vi "PSVCH_Caculate Thread.vi"() -> ()   [LabVIEW 2016]
uses:
  ShareLib/Formula/Ctrls/PSFormula_FOR_Formula Node.ctl
  ShareLib/Formula/Ctrls/PSFormula_FOR_Formula Step.ctl
  ShareLib/Formula/Ctrls/PSFormula_FOR_Formula Para.ctl
  ShareLib/Formula/Ctrls/PSFormula_FOR_Formula MidVar Data.ctl
  Ctrls/PSVCH_VarList.ctl
  <vilib>/Platform/TimedLoop/XDataNode/timing_clust.ctl
  <vilib>/Platform/TimedLoop/XDataNode/nitl_modes.ctl
  <vilib>/Platform/TimedLoop/XDataNode/wakeup.ctl
  <vilib>/Platform/TimedLoop/TimeConversion.llb/rt-timestamp-to-milliseconds.vi
  <vilib>/Pansino Software/LabVIEW Architecture/Queue Management/PSARC_Queue Insert Element.vi
  <vilib>/Platform/TimedLoop/XDataNode/XDataNode.xnode
  <vilib>/Platform/TimedLoop/XDataNode/XDNodeRunTimeDep.lvlib
  <vilib>/measure/NI_MABase.lvlib
panel:
  in  "Parameter":variant
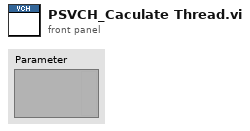
[diagram p1: front panel]
types:
  T1 = typedef "PSFormula_FOR_Formula Node.ctl" = cluster{"Formula Steps":T2[], "MidVar List":T4}
  T2 = typedef "PSFormula_FOR_Formula Step.ctl" = cluster{"Formula Calc":string, "Para":T3[], "Result Var":string, "Result Var Type":string}
  T3 = typedef "PSFormula_FOR_Formula Para.ctl" = cluster{"Para Index":i32, "Tag":string, "Type":string, "Label":string, "Data":variant}
  T4 = typedef "PSFormula_FOR_Formula MidVar Data.ctl" = cluster{"Names":string[], "Types":string[], "Values":variant[]}
  T5 = typedef "PSVCH_VarList.ctl" = cluster{"Tag[]":string[], "Type[]":string[], "Value[]":variant[], "ai[]":string[]}
  T6 = cluster{"Q_High Name":string, "字符串":string, "t0":timestamp, "Time":i64, "Exit":refnum<notifier>, "Dpl":refnum<queue>, "TDMS Ref":refnum<notifier>, "Save":refnum<notifier>, "Formula Node":T1, "VarList":T5, "布尔":bool, "字符串":string, "字符串":string}
  T7 = typedef "XDNodeRunTimeDep.lvlib/timing_clust.ctl" = cluster{"Expected End [f-1]":u64, "Actual End [f-1]":u64, "Finished Late? [f-1]":bool, "Expected End [i-1]":u64, "Actual End [i-1]":u64, "Finished Late? [i-1]":bool, "Expected Start [i]":u64, "Actual Start [i]":u64, "Expected Start [f]":u64, "Actual Start [f]":u64, "Source Name":string, "Structure Name":string, "Period":i64, "Deadline":i64, "Offset":i64, "Start":i64, "Priority":i32, "Timeout":i32, "Mode":T8, "Wakeup Reason":T9, "Error":errorcluster, "Source Type":string, "Secondary Source Type":string, "Global End Time":u64, "Global Start Time":u64, "Frame Duration":u64, "Iteration Duration":u64, "Assigned CPU":i32, "I/O Scan Engine Mode":u32}
  T8 = typedef "XDNodeRunTimeDep.lvlib/nitl_modes.ctl" = enum32{"No Change", "Process missed periods, maintain original phase", "Discard missed periods, maintain original phase", "Process missed periods, ignore original phase", "Discard missed periods, ignore original phase"}
  T9 = typedef "XDNodeRunTimeDep.lvlib/wakeup.ctl" = enum32{"Normal", "Aborted", "Asynchronous wakeup", "Timing source error", "Timed loop error", "Timeout"}
  T10 = cluster{"ai[]":string[], "Type[]":string[], "Value[]":variant[]}
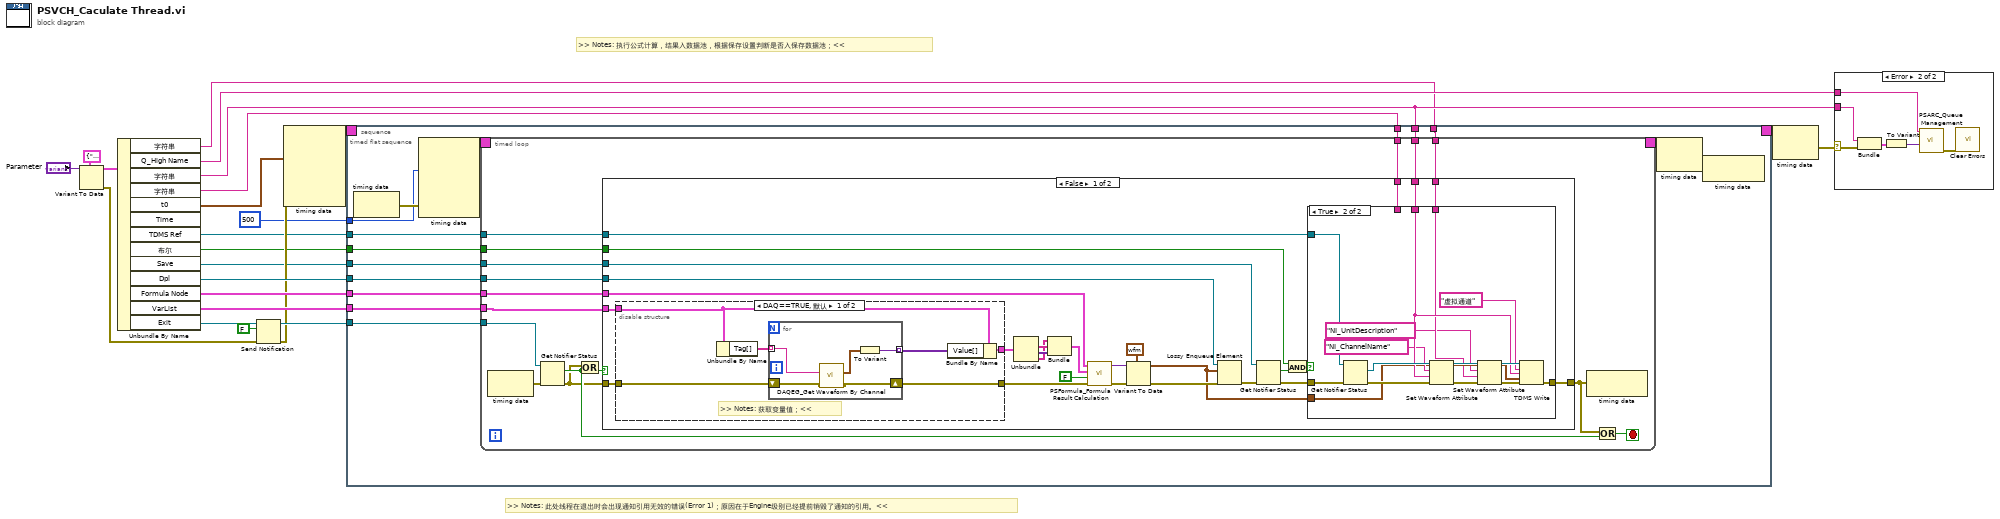
[diagram p0: block diagram]
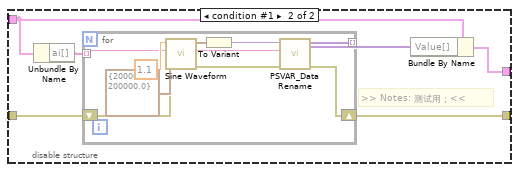
[diagram p3: hidden frame]
diagram:
  # ">> Notes: 此处线程在退出时会出现通知引用无效的错误(Error 1)；原因在于Engine级别已经提前销毁了通知的引用。<<"
  # ">> Notes: 执行公式计算，结果入数据池，根据保存设置判断是否入保存数据池；<<"
  n1 = Variant To Data(type=T6 {"Q_High Name"="", "字符串"="", "t0"=timestamp(0 s since 1904-01-01), "Time"=0, "Exit"=refnum, "Dpl"=refnum, "TDMS Ref"=refnum, "Save"=refnum, "Formula Node"={"Formula Steps"=[], "MidVar List"={"Names"=[], "Types"=[], "Values"=[]}}, "VarList"={"Tag[]"=[], "Type[]"=[], "Value[]"=[], "ai[]"=[]}, "布尔"=FALSE, "字符串"="", "字符串"=""} ("簇"), Variant="Parameter") -> (data=w23:T6, error out=w11:errorcluster)  [unwired: 1 in]
  n2 = Unbundle By Name(w23) -> ("字符串"=w3:string, "Q_High Name"=w21:string, "字符串"=w6:string, "字符串"=w4:string, "t0"=w14:timestamp, "TDMS Ref"=w8:refnum<notifier>, "布尔"=w5:bool, "Save"=w7:refnum<notifier>, "Dpl"=w20:refnum<queue>, "Formula Node"=w19:T1, "VarList"=w18:T5, "Exit"=w13:refnum<notifier>)  [unwired: 1 out]
  n3 = Send Notification(notification=FALSE ("通知"), notifier=w13, error in (no error)=w11) -> (notifier out=w12:refnum<notifier>, error out=w9:errorcluster)
  n4 = node-c288(w14, w9) -> (w17:T7)  [unwired: 3 in]
  n5 = timed-sequence {
    timing: w17 -> [_]
    timing-out: [_] -> w16
    tunnel: i64 500 ("Period") -> [w34]
    tunnel: w20 -> [w33]
    tunnel: w19 -> [w32]
    tunnel: w18 -> [w31]
    tunnel: w12 -> [w30]
    tunnel: w8 -> [w29]
    tunnel: w7 -> [w28]
    tunnel: w6 -> [w27]
    tunnel: w5 -> [w26]
    tunnel: w4 -> [w25]
    tunnel: w3 -> [w24]
    n6 = timed-flat-sequence {
      tunnel: w34 -> [w35]
      tunnel: w33 -> [w47]
      tunnel: w32 -> [w46]
      tunnel: w31 -> [w45]
      tunnel: w30 -> [w43]
      tunnel: w29 -> [w41]
      tunnel: w28 -> [w40]
      tunnel: w27 -> [w39]
      tunnel: w26 -> [w38]
      tunnel: w25 -> [w37]
      tunnel: w24 -> [w36]
      n7 = node-c288() -> (w42:errorcluster)  [unwired: 1 in]
      n8 = node-c288(w35, w42) -> (w49:T7)  [unwired: 3 in]
      n9 = timed-loop {
        timing: w49 -> [_]
        timing-out: [_] -> w48
        tunnel: w47 -> [w63]
        tunnel: w46 -> [w65]
        tunnel: w45 -> [w64]
        tunnel: w43 -> [w61]
        tunnel: w41 -> [w56]
        tunnel: w40 -> [w57]
        tunnel: w39 -> [w55]
        tunnel: w38 -> [w54]
        tunnel: w37 -> [w53]
        tunnel: w36 -> [w50]
        stop <- w58 stop-if-true
        n10 = node-c288() -> (w62:errorcluster)  [unwired: 1 in]
        n11 = Get Notifier Status(notifier=w61, error in (no error)=w62) -> (current notification=w59:bool, error out=w51:errorcluster)  [unwired: 3 out]
        n12 = Or(x=w51, y=w59) -> (x .or. y?=w52:bool)
        n13 = case shown="False" w52 {
          tunnel: w65 -> [w79 _]
          tunnel: w64 -> [w92 _]
          tunnel: [w86 w135] -> w60
          tunnel: w63 -> [w91 _]
          tunnel: w51 -> [w90 w135]
          tunnel: w57 -> [w88 _]
          tunnel: w56 -> [w85 _]
          tunnel: w55 -> [w84 _]
          tunnel: w54 -> [w82 _]
          tunnel: w53 -> [w80 _]
          tunnel: w50 -> [w67 _]
          frame False {
            n14 = disable-structure shown="DAQ==TRUE, 默认" {
              disable-tunnel: w92 -> [w114 w122]
              disable-tunnel: [w113 w125] -> w78
              disable-tunnel: w90 -> [w110 w124]
              disable-tunnel: [w109 w123] -> w71
              frame condition #0 (active) {
                # ">> Notes: 获取变量值；<<"
                n15 = Unbundle By Name(w114) -> ("Tag[]"=w111:string[])
                n16 = for {
                  tunnel: [w119] -> w112 mode=indexing
                  tunnel: w111 -> [w118] mode=indexing
                  shift-right: [w116] -> w109
                  shift-left: w110 -> [w117]
                  n17 = call "DAQEG_Get Waveform By Channel.vi"("error in (no error)"=w117, "DAQ Channel"=w118) -> ("error out"=w116:errorcluster, "waveform"=w115:waveform(dbl))  [unwired: 8 in]
                  n18 = To Variant(anything=w115) -> (Variant=w119:variant)
                }
                n19 = Bundle By Name(cluster=w114, "Value[]"=w112) -> (w113:T5)
              }
              frame condition #1 {
                # ">> Notes: 测试用；<<"
                n20 = Unbundle By Name(w122) -> ("ai[]"=w121:string[])
                n21 = for {
                  tunnel: [w129] -> w120 mode=indexing
                  tunnel: w121 -> [w126] mode=indexing
                  shift-right: [w127] -> w123
                  shift-left: w124 -> [w131]
                  n22 = call <vilib>:"Sine Waveform.vi"("sampling info"=cluster{"Fs":dbl, "#s":dbl} {"Fs"=200000.0, "#s"=200000.0}, "error in (no error)"=w131, "frequency"=1.1) -> ("error out"=w128:errorcluster, "signal out"=w132:waveform(dbl))  [unwired: 7 in]
                  n23 = To Variant(anything=w132) -> (Variant=w130:variant)
                  n24 = call <vilib>:"PSVAR_Data Rename.vi"("error in"=w128, "Name New"=w126, "Data In"=w130) -> ("error out"=w127:errorcluster, "Data Out"=w129:variant)  [unwired: 7 in]
                }
                n25 = Bundle By Name(cluster=w122, "Value[]"=w120) -> (w125:T5)
              }
            }
            n26 = Unbundle(w78) -> ("Type[]"=w77:string[], "Value[]"=w76:variant[], "ai[]"=w72:string[])  [unwired: 1 out]
            n27 = Bundle("ai[]"=w72, "Type[]"=w77, "Value[]"=w76) -> (w75:T10)  [unwired: 1 in]
            n28 = call "PSFormula_Formula Result Calculation.vi"("error in"=w71, "Complex Variable(T)"=FALSE, "Var List"=w75, "Formula Node"=w79) -> ("error out"=w70:errorcluster, "Result Value"=w74:variant)  [unwired: 5 in, 1 out]
            n29 = Variant To Data(error in=w70, type=waveform(dbl) {"t0"=timestamp(0 s since 1904-01-01), "dt"=1.0, "Y"=[]} ("Waveform"), Variant=w74) -> (data=w66:waveform(dbl), error out=w69:errorcluster)
            n30 = Lossy Enqueue Element(queue=w91, element=w66, error in (no error)=w69) -> (error out=w89:errorcluster)  [unwired: 3 out]
            n31 = Get Notifier Status(notifier=w88, error in (no error)=w89) -> (current notification=w83:bool, error out=w87:errorcluster)  [unwired: 3 out]
            n32 = And(x=w82, y=w83) -> (x .and. y?=w81:bool)
            n33 = case shown="True" w81 {
              tunnel: w87 -> [w93 w108]
              tunnel: [w93 w105] -> w86
              tunnel: w85 -> [_ w107]
              tunnel: w66 -> [_ w94]
              tunnel: w84 -> [_ w102]
              tunnel: w80 -> [_ _]
              tunnel: w67 -> [_ w96]
              frame False {
              }
              frame True {
                n34 = Get Notifier Status(notifier=w107, error in (no error)=w108) -> (current notification=w106:refnum<k34>, error out=w103:errorcluster)  [unwired: 3 out]
                n35 = Set Waveform Attribute(4:w103, 5:w102, 6:"NI_ChannelName" ("名称"), 7:w94) -> (0:w100:errorcluster, 3:w98:waveform(dbl))  [unwired: 1 out]
                n36 = Set Waveform Attribute(4:w100, 5:w96, 6:"NI_UnitDescription" ("名称"), 7:w98) -> (0:w99:errorcluster, 3:w97:waveform(dbl))  [unwired: 1 out]
                n37 = TDMS Write(0:w106, 5:"虚拟通道" ("组名称输入（无标题）"), 7:w102, 9:w97, 11:w99) -> (15:w105:errorcluster)  [unwired: 1 in, 3 out]
              }
            }
          }
          frame True {
          }
        }
        n38 = node-c288(w60) -> ()  [unwired: 1 out]
        n39 = Or(x=w60, y=w59) -> (x .or. y?=w58:bool)
      }
      n40 = node-c288(w48) -> (w44:errorcluster)
      n41 = node-c288(w44) -> ()  [unwired: 1 out]
    }
  }
  n42 = node-c288(w16) -> (w15:errorcluster)
  n43 = case shown="Error" w15 {
    selector: w15 -> [_ w156]
    tunnel: w21 -> [_ w154]
    tunnel: w6 -> [_ w152]
    frame No Error {
    }
    frame Error {
      n44 = Bundle("字符串"=w152, "error IO"=w156) -> (w155:cluster{"字符串":string, "error IO":errorcluster})  [unwired: 1 in]
      n45 = To Variant(anything=w155) -> (Variant=w157:variant)
      n46 = call-poly <vilib>:"PSARC_Queue Management.vi"("Data"=w157, "Queue Name(unamed)"=w154) -> ("error out"=w153:errorcluster)  [unwired: 8 in, 1 out]
      n47 = call <vilib>:"Clear Errors.vi"("error in (no error)"=w153) -> ()  [unwired: 5 in, 2 out]
    }
  }
